vi "post.vi"(7 "transmit queue":refnum<queue>, 10 "application request in":T1, 11 "test responder in":refnum<class "test responder.lvclass">) -> (0 "error out":errorcluster, 3 "test responder out":refnum<class "test responder.lvclass">)   [LabVIEW 2013, in "test responder.lvclass"]
uses:
  test responder.lvclass
  HTTP server/http response.ctl
  HTTP server/http response packet type.ctl
  HTTP headers/http header data.ctl
  HTTP server/http request.ctl
  HTTP server/http method.ctl
  HTTP responder/http responder.lvclass
  HTTP server/Basic HTTP server.lvclass
  HTTP headers/http headers.lvlib
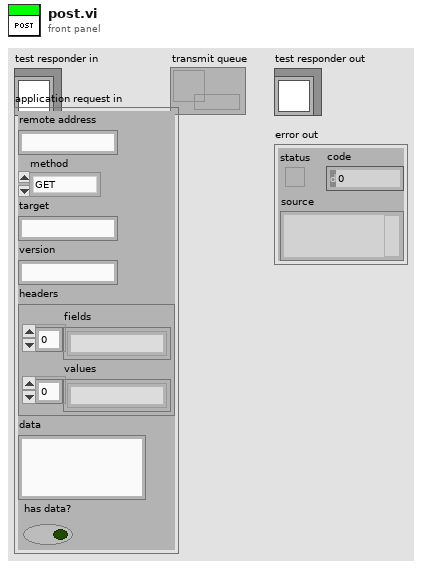
[diagram p1: front panel]
types:
  T1 = typedef "Basic HTTP server.lvclass/http request.ctl" = cluster{"remote address":string, "method":T2, "target":string, "version":string, "headers":T3, "data":string, "has data?":bool}
  T2 = typedef "Basic HTTP server.lvclass/http method.ctl" = enum16{"GET", "POST", "PUT", "DELETE", "HEAD", "OPTIONS", "upgrade"}
  T3 = typedef "http headers.lvlib/http header data.ctl" = cluster{"fields":string[], "values":string[]}
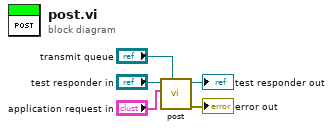
[diagram p0: block diagram]
diagram:
  n1 = call-parent "post.vi"("transmit queue"="transmit queue", "application request in"="application request in", "http responder in"="test responder in") -> ("error out"=→"error out":errorcluster, "http responder out"=→"test responder out":refnum<class "test responder.lvclass">)  [unwired: 7 in]
